vi "InitDGObj and HW from CnfgFile.vi"(4 "error in":errorcluster, 7 "BME_DG_System in":refnum<class "BME_DG_System.lvclass">) -> (0 "error IO":errorcluster, 3 "BME_DG_System Out":refnum<class "BME_DG_System.lvclass">)   [LabVIEW 2009, in "POLARIS BME DG.lvlib" / "BME_DG_System.lvclass"]
uses:
  BME_DG_System.lvclass
  BME_DG_System.lvclass/BME_DG_System.ctl
  POLARIS BME DG.lvlib
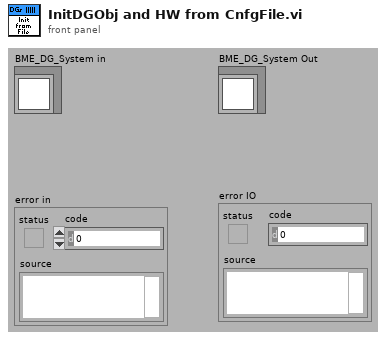
[diagram p1: front panel]
types:
  T1 = typedef "POLARIS BME DG.lvlib/System DG Selection.ctl" = cluster{"Selected System DGs":T2[], "Name":string}
  T2 = typedef "POLARIS BME DG.lvlib/DetectDG.ctl" = cluster{"DG_Number":i32, "DG_Product":i32, "Product Name":string, "Bus_Number":i32, "Slot_Number":i32, "Master":bool}
  T3 = typedef "POLARIS BME DG.lvlib/Card Config.ctl" = cluster{"Logical Name":string, "Base Settings":T4, "SG08_Settings":T6, "Channel Names":string[], "Advanced Settings":T7}
  T4 = typedef "POLARIS BME DG.lvlib/BME_DG_TriggerSettings.ctl" = cluster{"Clock Source":T5, " clock modulo":u32, "TriggerEnabled?":bool, "trigger modulo ":i32, "InputTerminated?":bool, "Inhibit(µs)":dbl, "TriggerLevel":dbl, "PresetValue":i32, "InternalTrigger?":bool, "InternalArm?":bool, "SWTrigger?":bool, "RisingEdge?":bool, "StopOnPreset?":bool, "ResetWhenDone?":bool, "Gate Divider":i32, "PositiveGate?":bool}
  T5 = typedef "POLARIS BME DG.lvlib/ClockSource.ctl" = i32
  T6 = typedef "POLARIS BME DG.lvlib/SG08_Settings.ctl" = cluster{"Gate Terminate":bool, "Gate Level":dbl, "Gate Delay (µs)":dbl, "StepBackTime (µs)":dbl, "Burst Counter":u32, "Trigger Divider":u32, "Trigger Multiplier":u32}
  T7 = typedef "POLARIS BME DG.lvlib/BME_DG_V2TriggerSettings.ctl" = cluster{"Trigger on MS Bus":T8, "Force Trigger (µs)":dbl, "Gate Type":bool, "Synchronize Gate":bool}
  T8 = typedef "POLARIS BME DG.lvlib/MSBus.ctl" = u32
  T9 = typedef "POLARIS BME DG.lvlib/Chnl Settings Complete.ctl" = cluster{"Channel Name":string, "ChnParameter":T10, "DelayFormula":string, "OutputModulo":i32, "Go and Done Signal":T11, "G08_Chnl_Settings":T12}
  T10 = typedef "POLARIS BME DG.lvlib/ChnlSettings.ctl" = cluster{" Delay (µs)":dbl, "On?":bool, "PositiveVoltage?":bool, "50OhmTerminated? ":bool, "25OhmOutput?":bool}
  T11 = typedef "POLARIS BME DG.lvlib/Go_Done_Chnl_Settings.ctl" = cluster{"Go Signal":T8, "Done Signal":u32}
  T12 = typedef "POLARIS BME DG.lvlib/SG08_Chnl_Settings.ctl" = cluster{"Pulse Width (µs)":dbl, "Output Offset":u32, "Disconnect (E,F)":bool, "Onto MsBus (E,F)":bool, "Input Positive (E,F)":bool}
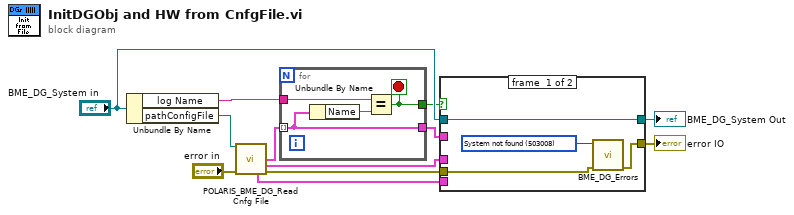
[diagram p0: block diagram]
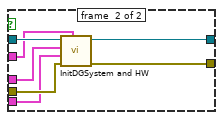
[diagram p2: hidden frame]
diagram:
  n1 = Unbundle By Name("BME_DG_System in") -> ("log Name"=w11:string, "pathConfigFile"=w8:path)
  n2 = call "POLARIS_BME_DG_Read Cnfg File.vi"("Config File"=w8, "error in (no error)"="error in") -> ("DGSystems"=w5:T1[], "Cards"=w4:T3[], "Chnls"=w3:T9[], "error out"=w6:errorcluster)  [unwired: 8 in, 2 out]
  n3 = for {
    tunnel: w5 -> [w13] mode=indexing
    tunnel: w11 -> [w14]
    tunnel: [w15] -> w10
    tunnel: [w13] -> w9
    stop <- w15 stop-if-true
    n4 = Unbundle By Name(w13) -> ("Name"=w16:string)
    n5 = Equal?(x=w14, y=w16) -> (x = y?=w15:bool)
  }
  n6 = case shown="True" w10 {
    tunnel: [w18 w21] -> w1
    tunnel: [w20 w22] -> w2
    tunnel: w6 -> [w19 w25]
    tunnel: "BME_DG_System in" -> [w20 w27]
    tunnel: w9 -> [_ w26]
    tunnel: w4 -> [_ w24]
    tunnel: w3 -> [_ w23]
    frame #0 {
      w17 = 503008 items=["Channel refers itself"=503001, "Deadloop"=503002, "Negative Delay"=503003, "Delay Card not found"=503004, "Channel not found"=503005, "Parse Error"=503006, "Not Supported"=503007, "System not found"=503008] ("error")
      n7 = call "BME_DG_Errors.vi"("error in (no error)"=w19, "error"=w17) -> ("error out"=w18:errorcluster)  [unwired: 9 in]
    }
    frame #1 {
      n8 = call "InitDGSystem and HW.vi"("System"=w26, "error in"=w25, "Chnls"=w23, "Cards"=w24, "BME_DG_System in"=w27) -> ("error out"=w21:errorcluster, "BME_DG_System in"=w22:refnum<class "BME_DG_System.lvclass">)  [unwired: 4 in, 1 out]
    }
  }
  "error IO" <- w1
  "BME_DG_System Out" <- w2
